vi "Set Windows Desktop Background Image LabVIEW 2013 NIVerified.vi"(8 "error in (no error)":errorcluster, 11 "Path":path) -> (0 "error out":errorcluster)   [LabVIEW 2020]
doc: "This example uses the Windows API to programatically set the the desktop wallpaper image. This program uses the user32.dll and the SystemParameeresInfoA function to set the background image."
uses:
  Windows/System32/user32.dll
panel:
  # "Overview: This example uses the Windows API to programmatically set the the desktop wallpaper image.\nRequirements: LabVIEW 2013 (or compatible).\nInstructions:\n1. Simply select a path to an image and run the code.\n2. The background with change to the image you selected."
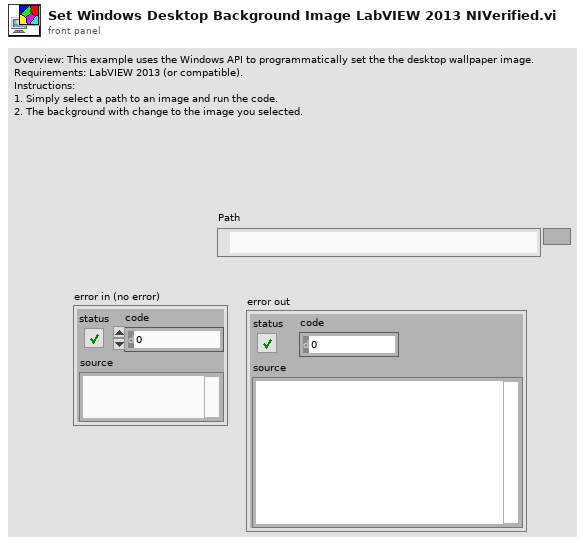
[diagram p1: front panel]
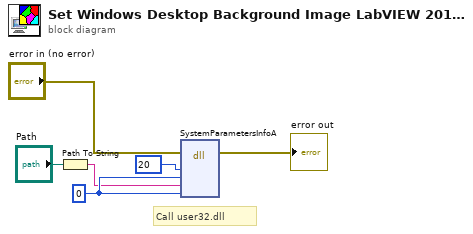
[diagram p0: block diagram]
diagram:
  w5 = u32 0 ("uiParam")
  # "Call user32.dll"
  n1 = Path To String(path="Path") -> (string=w3:string)
  n2 = dll-call lib="/Windows/System32/user32.dll" fn="SystemParametersInfoA"(error in="error in (no error)", "uiAction"=u32 20, "uiParam"=w5, "pvParam"=w3, "fWinINI"=w5) -> (error out=→"error out":errorcluster)  [unwired: 7 in, 1 out]
